vi "Specified_Channels_client.vi"(6 "Mode":T1, 9 "End time":dbl, 10 "Start time":dbl, 11 "ADAM Index array":i32[](array[numeric])) -> (0 "Output array":dbl[][](array[numeric]) format="%.2f", 1 "Averaging Period":dbl[](array[numeric]) format="%.2f", 2 "Centre Times":dbl[](array[numeric]) format="%.2f", 3 "All Active Ch Names":string[](array[string]), 4 "Messages":string)   [LabVIEW 2020]
doc: "This is an example of using features of the VI Server as a client. It shows how you might browse from one or more applications that may be exporting data from one or more data stations. \n\nThe example shows how to query a server for its list of exported VIs, how to get references to the VIs, and how call them with the Call By Reference function."
uses:
  Sub VIs/ADAM Controls/Search_mode.ctl
  Anemometry/Anemometry Sub Vis/Controls/Server_Comms.ctl
  Anemometry/Anemometry Sub Vis/Globals/Preference_global.vi
panel:
  in  "vi type":refnum<vi>
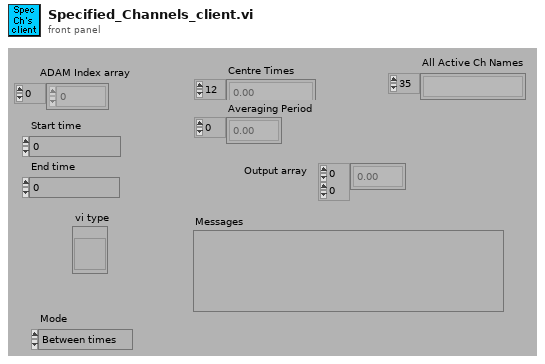
[diagram p1: front panel]
types:
  T1 = typedef "Search_mode.ctl" = enum16{"Between times", "All Times"}
  T2 = typedef "Server_Comms.ctl" = enum16{"Do Not Link To Server", "Server Link Healthy"}
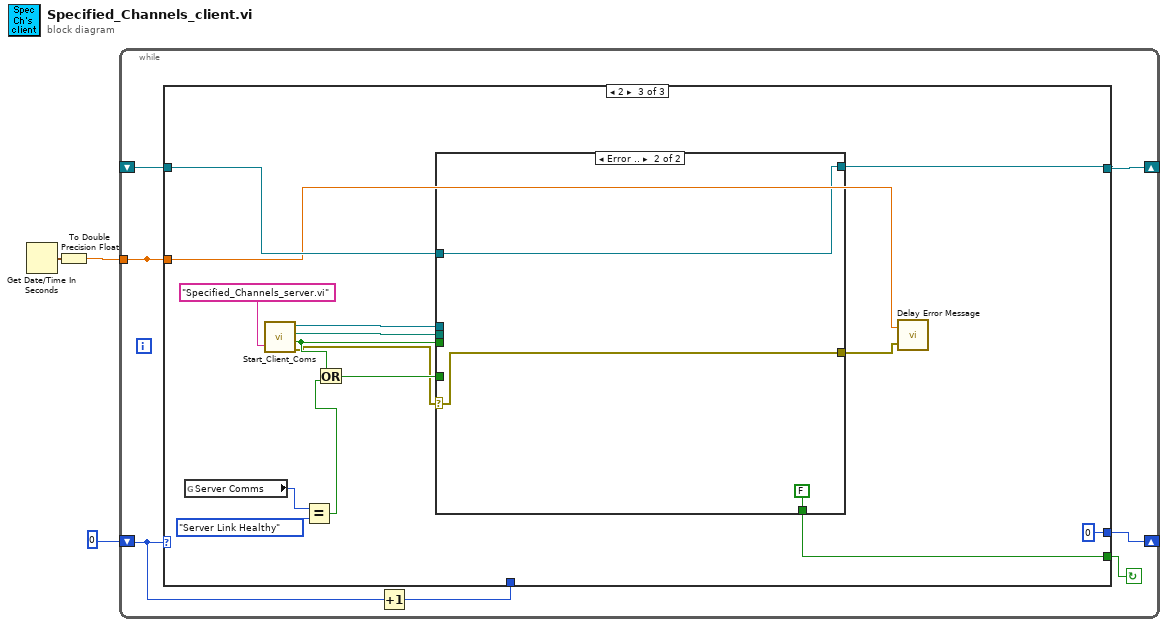
[diagram p0: block diagram]
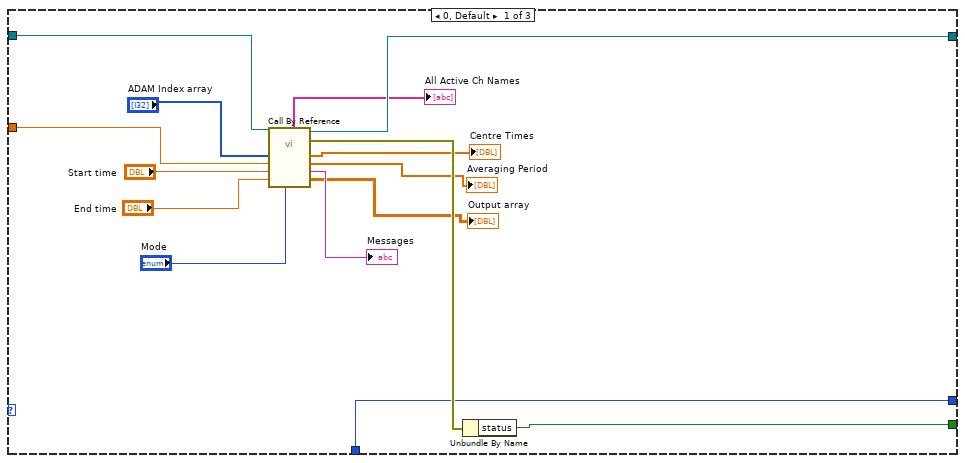
[diagram p2: hidden frame]
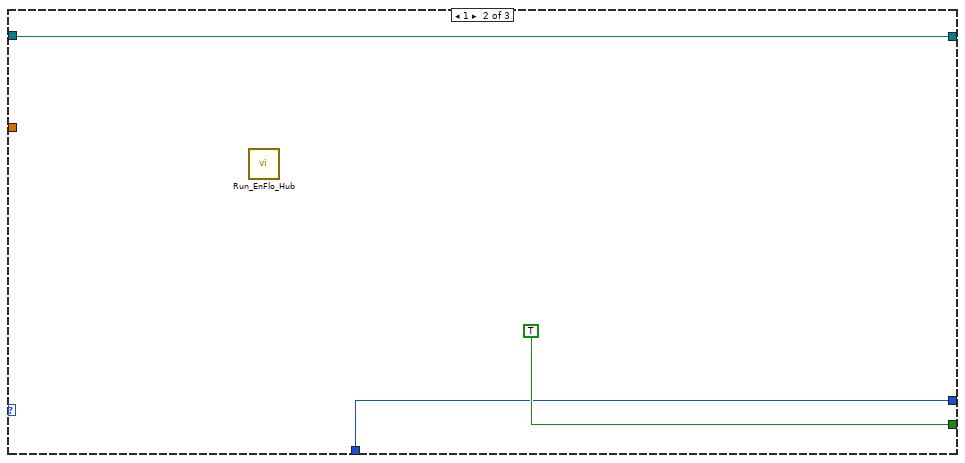
[diagram p3: hidden frame]
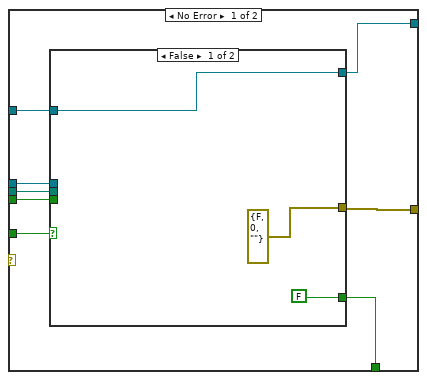
[diagram p4: hidden frame]
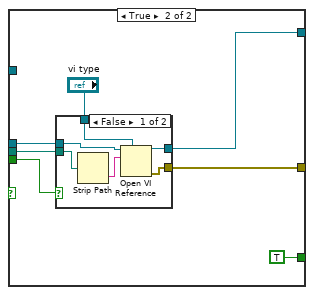
[diagram p5: hidden frame]
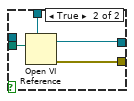
[diagram p6: hidden frame]
diagram:
  n1 = Get Date/Time In Seconds() -> (seconds since 1Jan1904=w2:timestamp)
  n2 = To Double Precision Float(number=w2) -> (double precision float=w1:dbl)
  n3 = while {
    shift-left: 0 -> [w7]
    shift-right: [w5] -> _
    shift-left: _ -> [w9]
    shift-right: [w10] -> _
    tunnel: w1 -> [w6]
    tunnel: [w6] -> _
    stop <- w4 continue-if-true
    n4 = Increment(x=w7) -> (x+1=w8:i32)
    n5 = case shown="2" w7 {
      tunnel: [w20 w28 w43] -> w10
      tunnel: [w18 TRUE ("status") w33] -> w4
      tunnel: w9 -> [w21 w28 w34]
      tunnel: w8 -> [w11 w26 _]
      tunnel: w6 -> [w12 _ w30]
      tunnel: [w11 w26 0] -> w5
      frame 0, Default {
        n6 = call-by-ref "?"(reference=w21, "Mode"="Mode", "End time"="End time", "Start time"="Start time", "Clients time"=w12, "Requested channels"="ADAM Index array") -> (reference out=w20:refnum<vi>, error out=w19:errorcluster, "Output array"=→"Output array":dbl[][], "Messages"=→"Messages":string, "Averaging Period"=→"Averaging Period":dbl[], "Centre Times"=→"Centre Times":dbl[], "All Active Ch Names"=→"All Active Ch Names":string[])  [unwired: 1 in]
        n7 = Unbundle By Name(w19) -> ("status"=w18:bool)
      }
      frame 1 {
        n8 = call "Run_EnFlo_Hub.vi"() -> ()  [unwired: 1 in, 7 out]
      }
      frame 2 {
        n9 = global read "Preference_global.vi" "Server Comms"() -> (w38:T2)
        n10 = call "Start_Client_Coms.vi"("VI name to run on server"="Specified_Channels_server.vi") -> ("LabVIEW application reference"=w40:refnum<vi>, "Checked VI name"=w41:path, "Local Call"=w36:bool, "Error cluster"=w29:errorcluster)  [unwired: 1 in]
        n11 = Equal?(x=w38, y=Server_Comms."Server Link Healthy" ("Server Comms")) -> (x = y?=w37:bool)
        n12 = Or(x=w36, y=w37) -> (x .or. y?=w35:bool)
        n13 = case shown="Error .." w29 {
          selector: w29 -> [_ w73]
          tunnel: [w51 w72] -> w43
          tunnel: w41 -> [w50 _]
          tunnel: w40 -> [w49 _]
          tunnel: w36 -> [w48 _]
          tunnel: w35 -> [w47 _]
          tunnel: w34 -> [w46 w72]
          tunnel: [w45 FALSE ("status")] -> w33
          tunnel: [w44 w73] -> w31
          frame No Error {
            n14 = case shown="False" w47 {
              tunnel: [w53 w61] -> w51
              tunnel: [errorcluster {"status"=FALSE, "code"=0, "source"=""} ("error out") w56] -> w44
              tunnel: w50 -> [_ w60]
              tunnel: w49 -> [_ w59]
              tunnel: w48 -> [_ w58]
              tunnel: w46 -> [w53 _]
              tunnel: [FALSE ("status") TRUE ("status")] -> w45
              frame False {
              }
              frame True {
                n15 = case shown="False" w58 {
                  tunnel: [w66 w71] -> w61
                  tunnel: "vi type" -> [w63 w70]
                  tunnel: w60 -> [w64 w69]
                  tunnel: w59 -> [w62 _]
                  tunnel: [w65 w68] -> w56
                  frame False {
                    n16 = Strip Path(path=w64) -> (name=w67:string)  [unwired: 1 out]
                    n17 = Open VI Reference(type specifier VI Refnum (for type only)=w63, application reference (local)=w62, vi path=w67) -> (vi reference=w66:refnum<vi>, error out=w65:errorcluster)  [unwired: 1 in, 2 out]
                  }
                  frame True {
                    n18 = Open VI Reference(type specifier VI Refnum (for type only)=w70, vi path=w69) -> (vi reference=w71:refnum<vi>, error out=w68:errorcluster)  [unwired: 1 in, 3 out]
                  }
                }
              }
            }
          }
          frame Error {
          }
        }
        n19 = call "Delay Error Message.vi"("error in (no error)"=w31, "Seconds since 1904"=w30) -> ()  [unwired: 2 in]
      }
    }
  }
